vi "Initial_Simplex_Amplitude_v2.vi"(1 "Zernike Modes 3":i32[](array[numeric])=[5, 6, 7, 8], 2 "Depth (um)":dbl format="%#_13g", 3 "Zernike Modes 2":i32[](array[numeric])=[5, 6, 7, 8], 4 "Slope":path=path "C:/Users/Mlodzianoski/Desktop/Microscope 2 Labview Programs/VIs/DM/Mike/FitVal_ZMode_Depth_Corr2.txt", 5 "Zernike Modes 1":i32[](array[numeric])=[11, 22], 6 "Aberration Correction Choice":u16(ring) items=["Spherical Aberrations", "Astigmatism", "Coma"]) -> (0 "Initial Simplex Amplitude":dbl[][](array[numeric]))   [LabVIEW 2015]
uses:
  <vilib>/Utility/file.llb/Read Delimited Spreadsheet (DBL).vi
panel:
  in  "Factional Change":dbl=0.5 format="%#_13g"
  in  "Manual Inputs":dbl[](array[numeric])=[0.0, 0.0, 0.0, 0.0, 0.1, 0.1, -0.2, -0.2, 0.0, 0.0, -0.5, 0.0, 0.0, 0.0, 0.0, 0.0, 0.0, 0.0, 0.0, 0.0, 0.0, -0.2]
  in  "Read from File":bool=TRUE
  in  "Multiple Input Params per Zernike Mode":bool
  in  "Input Change":dbl=0.5 format="%#_13g"
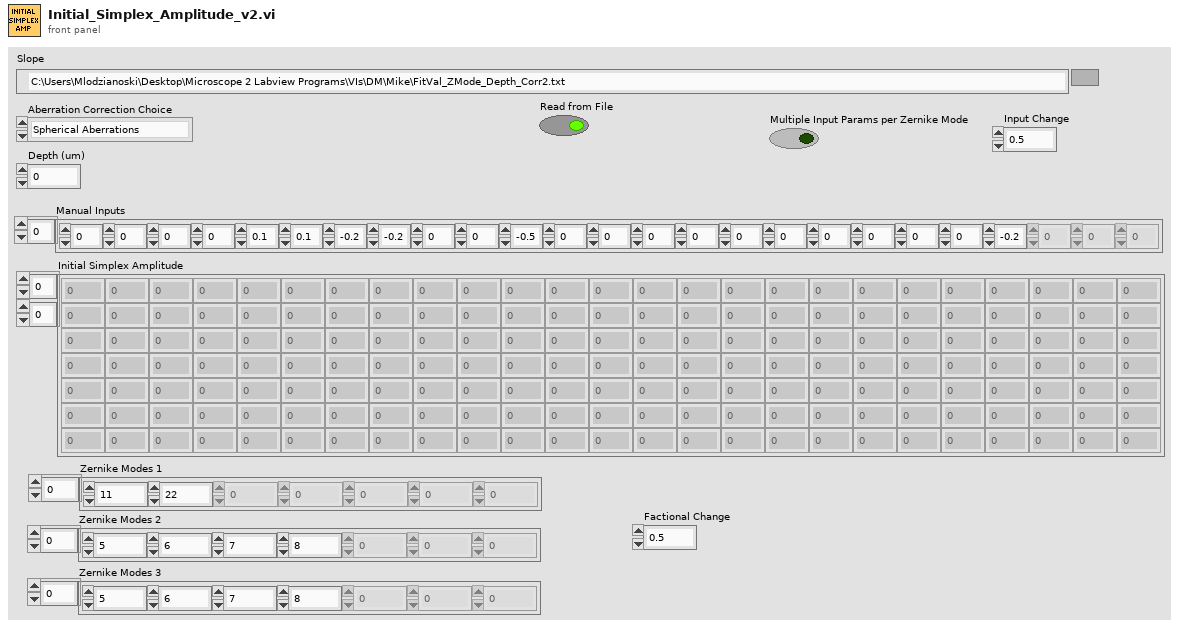
[diagram p1: front panel]
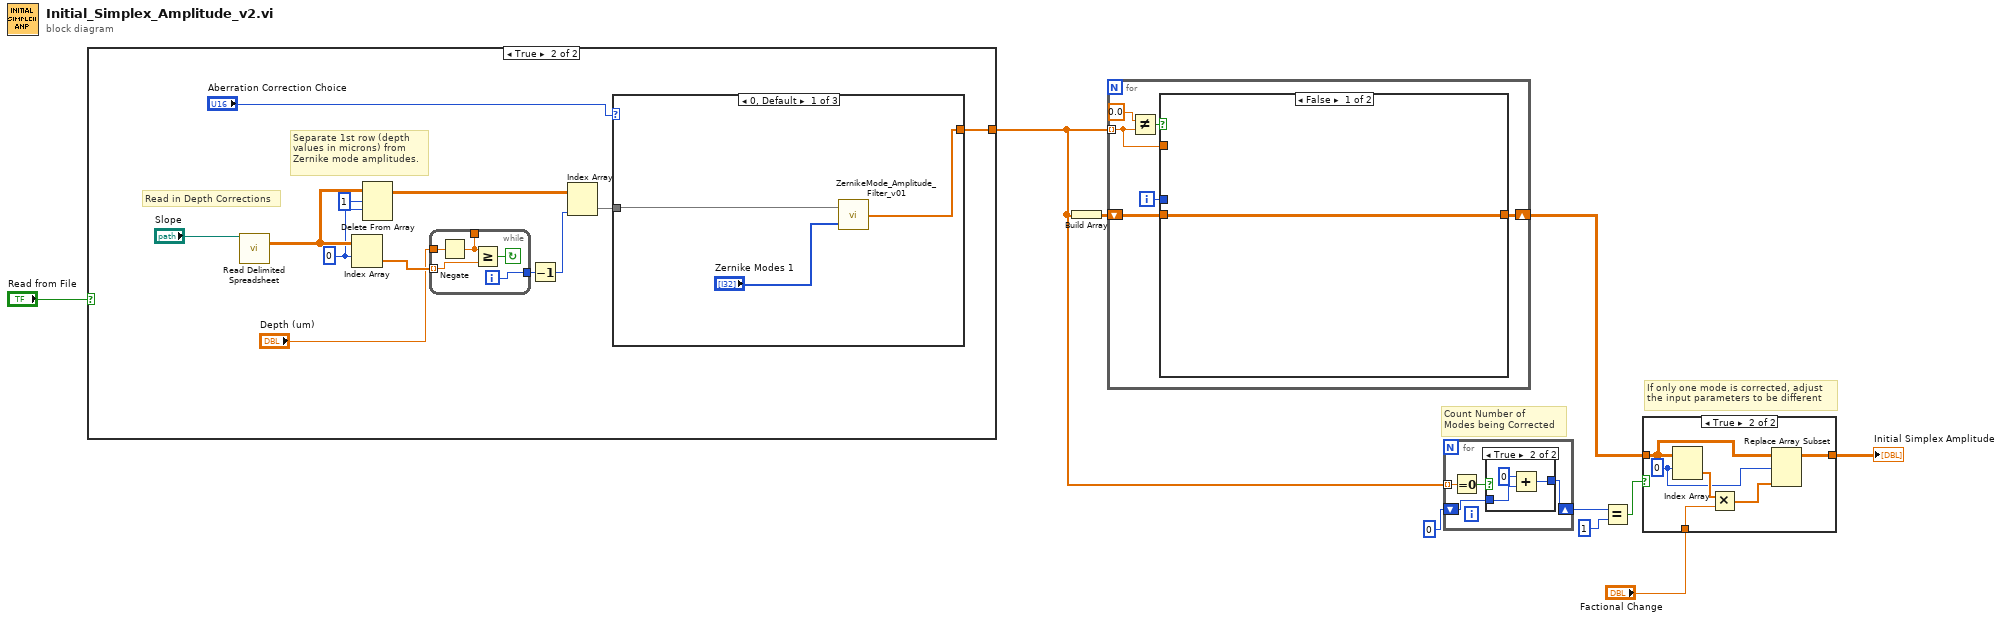
[diagram p0: block diagram]
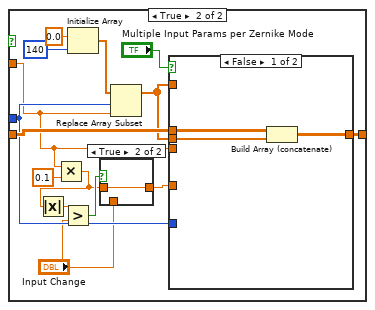
[diagram p3: hidden frame]
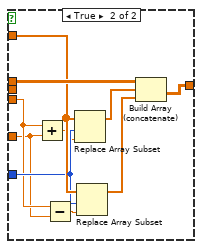
[diagram p5: hidden frame]
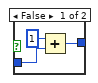
[diagram p6: hidden frame]
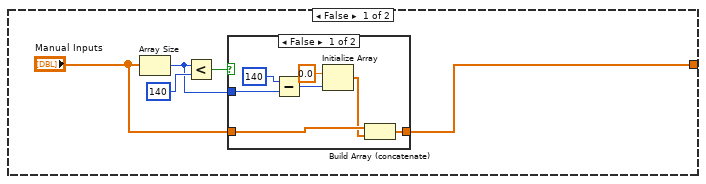
[diagram p7: hidden frame]
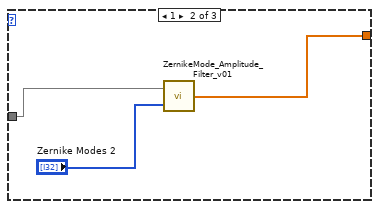
[diagram p9: hidden frame]
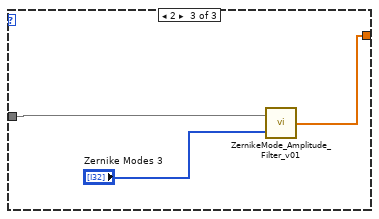
[diagram p10: hidden frame]
diagram:
  # "If only one mode is corrected, adjust \nthe input parameters to be different"
  # "Count Number of \nModes being Corrected"
  n1 = case shown="True" "Read from File" {
    tunnel: [w12 w25] -> w9
    frame False {
      n2 = Array Size(array="Manual Inputs") -> (size(s)=w11:i32)
      n3 = Less?(x=w11, y=140) -> (x < y?=w14:bool)
      n4 = case shown="False" w14 {
        tunnel: "Manual Inputs" -> [w18 w23]
        tunnel: [w16 w23] -> w12
        tunnel: w11 -> [w20 _]
        frame False {
          n5 = Subtract(x=140 ("dimension size"), y=w20) -> (x-y=w19:i32)
          n6 = Initialize Array(0.0 ("element"), w19) -> (w17:dbl[])
          n7 = Build Array (concatenate)(w18, w17) -> (w16:dbl[])
        }
        frame True {
        }
      }
    }
    frame True {
      w26 = 0 ("index (row)")
      # "Separate 1st row (depth \nvalues in microns) from \nZernike mode amplitudes."
      # "Read in Depth Corrections"
      n8 = call-poly <vilib>:"Read Delimited Spreadsheet.vi"("file path (dialog if empty)"="Slope") -> ("all rows"=w29:dbl[][])  [unwired: 9 in, 5 out]
      n9 = Index Array(array=w29, index (row)=w26) -> (element=w31:dbl[])  [unwired: 1 in]
      n10 = Delete From Array(array=w29, length=1, index (row)=w26) -> (array with subset deleted=w33:dbl[][])  [unwired: 1 in, 1 out]
      n11 = while {
        tunnel: "Depth (um)" -> [w37]
        tunnel: w31 -> [w38] mode=indexing
        tunnel: [w39] -> w32
        tunnel: [w36] -> _
        i -> [w39]
        stop <- w40 continue-if-true
        n12 = Negate(x=w37) -> (-x=w36:dbl)
        n13 = Greater Or Equal?(x=w36, y=w38) -> (x >= y?=w40:bool)
      }
      n14 = Decrement(x=w32) -> (x-1=w34:i32)
      n15 = Index Array(array=w33, index (col)=w34) -> (element=w35:dbl[])  [unwired: 1 in]
      n16 = case shown="0, Default" "Aberration Correction Choice" {
        tunnel: w35 -> [w42 w46 w48]
        tunnel: [w41 w45 w47] -> w25
        frame 0, Default {
          n17 = call "ZernikeMode_Amplitude_Filter_v01.vi"("Zernike Modes"="Zernike Modes 1", "Zernike Mode Amp Guess Input"=w42) -> ("Zernike Modes Amplitudes Output"=w41:dbl[])
        }
        frame 1 {
          n18 = call "ZernikeMode_Amplitude_Filter_v01.vi"("Zernike Modes"="Zernike Modes 2", "Zernike Mode Amp Guess Input"=w46) -> ("Zernike Modes Amplitudes Output"=w45:dbl[])
        }
        frame 2 {
          n19 = call "ZernikeMode_Amplitude_Filter_v01.vi"("Zernike Modes"="Zernike Modes 3", "Zernike Mode Amp Guess Input"=w48) -> ("Zernike Modes Amplitudes Output"=w47:dbl[])
        }
      }
    }
  }
  n20 = Build Array(w9) -> (w5:dbl[][])
  n21 = for {
    tunnel: w9 -> [w53] mode=indexing
    shift-right: [w51] -> w3
    shift-left: w5 -> [w50]
    i -> [w52]
    n22 = Not Equal?(x=0.0 ("y"), y=w53) -> (x != y?=w55:bool)
    n23 = case shown="False" w55 {
      tunnel: w53 -> [_ w63]
      tunnel: w52 -> [_ w66]
      tunnel: [w56 w68] -> w51
      tunnel: w50 -> [w56 w67]
      frame False {
      }
      frame True {
        n24 = Multiply(x=w63, y=0.1) -> (x*y=w57:dbl)
        n25 = Absolute Value(x=w57) -> (abs(x)=w58:dbl)
        n26 = Greater?(x=w58, y="Input Change") -> (0:w61:bool)
        n27 = Initialize Array(0.0 ("element"), 140 ("dimension size")) -> (w69:dbl[])
        n28 = case shown="True" w61 {
          tunnel: [w72 w73] -> w60
          tunnel: w57 -> [_ w73]
          tunnel: "Input Change" -> [w72 _]
          frame False {
          }
          frame True {
          }
        }
        n29 = Replace Array Subset(array=w69, new element=w63, index=w66) -> (w65:dbl[])
        n30 = case shown="False" "Multiple Input Params per Zernike Mode" {
          tunnel: w65 -> [w76 _]
          tunnel: [w75 w85] -> w68
          tunnel: w67 -> [w74 w86]
          tunnel: w66 -> [_ w82]
          tunnel: w65 -> [_ w83]
          tunnel: w63 -> [_ w79]
          tunnel: w60 -> [_ w77]
          frame False {
            n31 = Build Array (concatenate)(w74, w76) -> (w75:dbl[][])
          }
          frame True {
            n32 = Add(x=w79, y=w77) -> (x+y=w80:dbl)
            n33 = Subtract(x=w79, y=w77) -> (x-y=w78:dbl)
            n34 = Replace Array Subset(array=w83, new element=w80, index=w82) -> (w84:dbl[])
            n35 = Replace Array Subset(array=w83, new element=w78, index=w82) -> (w81:dbl[])
            n36 = Build Array (concatenate)(w86, w84, w81) -> (w85:dbl[][])
          }
        }
      }
    }
  }
  n37 = for {
    tunnel: w9 -> [w90] mode=indexing
    shift-right: [w88] -> w7
    shift-left: 0 -> [w87]
    n38 = Equal To 0?(x=w90) -> (x = 0?=w89:bool)
    n39 = case shown="True" w89 {
      tunnel: [w92 w95] -> w88
      tunnel: w87 -> [w93 w96]
      frame False {
        n40 = Add(x=1, y=w93) -> (x+y=w92:i32)
      }
      frame True {
        n41 = Add(x=0, y=w96) -> (x+y=w95:i32)
      }
    }
  }
  n42 = Equal?(x=w7, y=1) -> (x = y?=w4:bool)
  n43 = case shown="True" w4 {
    tunnel: w3 -> [w97 w102]
    tunnel: [w97 w99] -> w2
    tunnel: "Factional Change" -> [_ w98]
    frame False {
    }
    frame True {
      w101 = 0 ("index (row)")
      n44 = Index Array(array=w102, index (row)=w101) -> (element=w103:dbl[])  [unwired: 1 in]
      n45 = Multiply(x=w103, y=w98) -> (x*y=w100:dbl[])
      n46 = Replace Array Subset(array=w102, new element=w100, index (row)=w101) -> (w99:dbl[][])  [unwired: 1 in]
    }
  }
  "Initial Simplex Amplitude" <- w2
